vi "Get First Diagonal Recursively.vi"(10 "Data":i64[](array[numeric]), 11 "Result":i64[](array[numeric])) -> (3 "Array":i64[](array[numeric]))   [LabVIEW 2020, in "Measurement.lvclass"]
uses:
  Measurement.lvclass
  Measurement.lvclass/Measurement.ctl
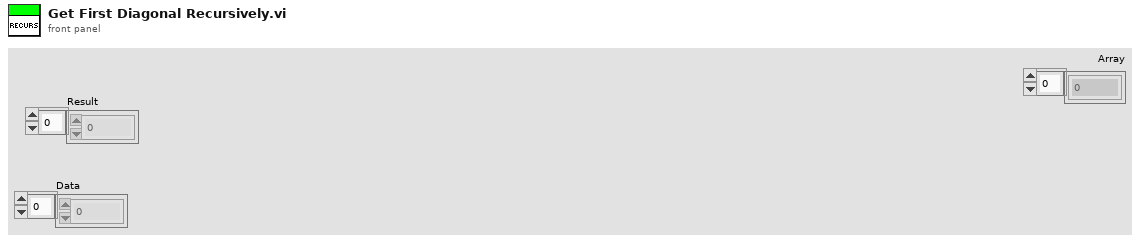
[diagram p1: front panel]
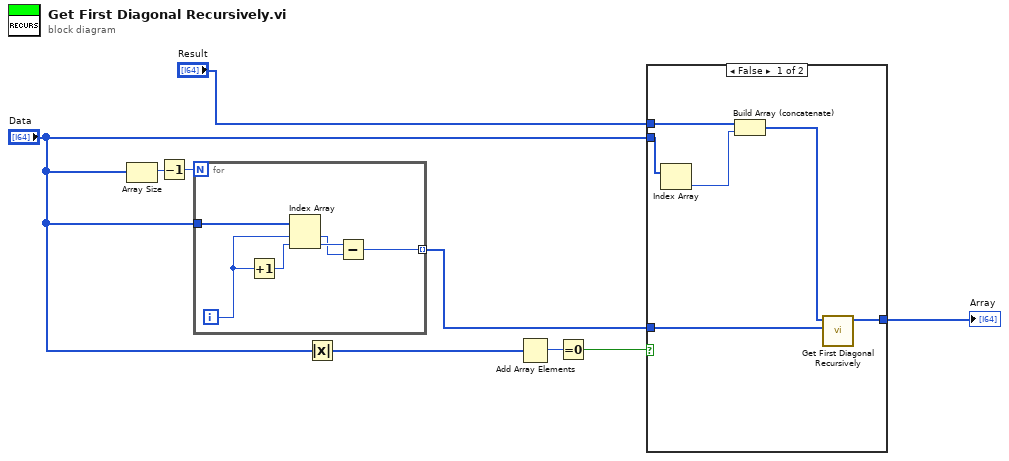
[diagram p0: block diagram]
diagram:
  n1 = Array Size(array="Data") -> (size(s)=w8:i32)
  n2 = Decrement(x=w8) -> (x-1=w9:i32)
  n3 = for {
    N: w9 -> [_]
    tunnel: "Data" -> [w15]
    tunnel: [w10] -> w3 mode=indexing
    i -> [w13]
    n4 = Increment(x=w13) -> (x+1=w14:i32)
    n5 = Index Array(array=w15, index #1=w13, index #2=w14) -> (element #1=w11:i64, element #2=w12:i64)
    n6 = Subtract(x=w12, y=w11) -> (x-y=w10:i64)
  }
  n7 = Absolute Value(x="Data") -> (abs(x)=w5:i64[])
  n8 = Add Array Elements(numeric array=w5) -> (sum=w7:i64)
  n9 = Equal To 0?(x=w7) -> (x = 0?=w6:bool)
  n10 = case shown="False" w6 {
    tunnel: w3 -> [w21 _]
    tunnel: [w20 w22] -> w4
    tunnel: "Result" -> [w18 w22]
    tunnel: "Data" -> [w17 _]
    frame False {
      n11 = Index Array(array=w17) -> (element=w19:i64)  [unwired: 1 in]
      n12 = Build Array (concatenate)(w18, w19) -> (w16:i64[])
      n13 = call "Get First Diagonal Recursively.vi"("Data"=w21, "Result"=w16) -> ("Array"=w20:i64[])  [unwired: 9 in]
    }
    frame True {
    }
  }
  "Array" <- w4
